vi "Practica 8 - Compuertas Logicas.vi"() -> ()   [LabVIEW 2023]
panel:
  out "XOR":bool
  out "NOR":bool
  out "NAND":bool
  out "NOT":bool
  out "OR":bool
  out "AND":bool
  in  "B":bool
  in  "A":bool
  # "COMPUERTAS LOGICAS"
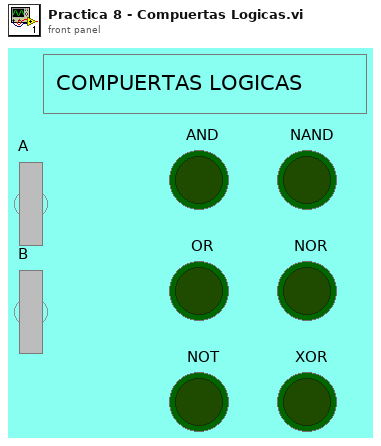
[diagram p1: front panel]
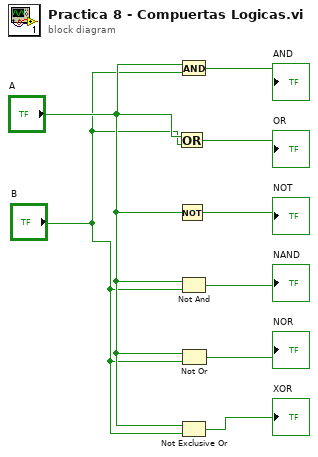
[diagram p0: block diagram]
diagram:
  n1 = Or(x="A", y="B") -> (x .or. y?=→"OR":bool)
  n2 = Not(x="A") -> (.not. x?=→"NOT":bool)
  n3 = And(x="A", y="B") -> (x .and. y?=→"AND":bool)
  n4 = Not And(1:"B", 2:"A") -> (0:→"NAND":bool)
  n5 = Not Or(1:"B", 2:"A") -> (0:→"NOR":bool)
  n6 = Not Exclusive Or(1:"B", 2:"A") -> (0:→"XOR":bool)
